vi "Replace Row In File.vi"(9 "Index":i32, 10 "Insert Array":dbl[](array[numeric]), 11 "Path":path) -> (0 "error out":errorcluster)   [LabVIEW 2016]
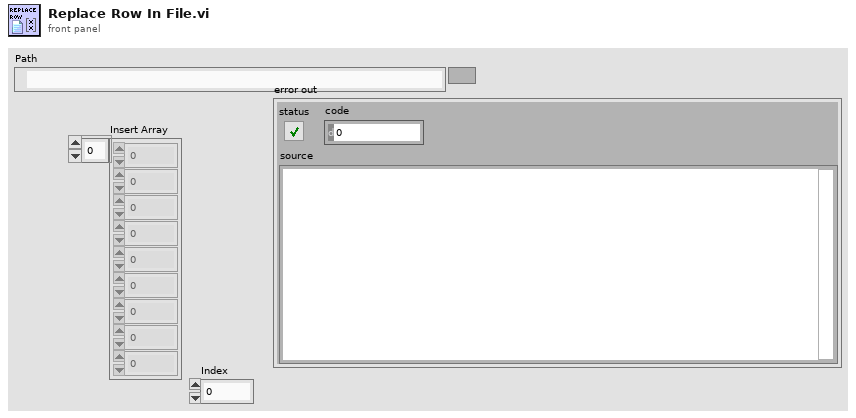
[diagram p1: front panel]
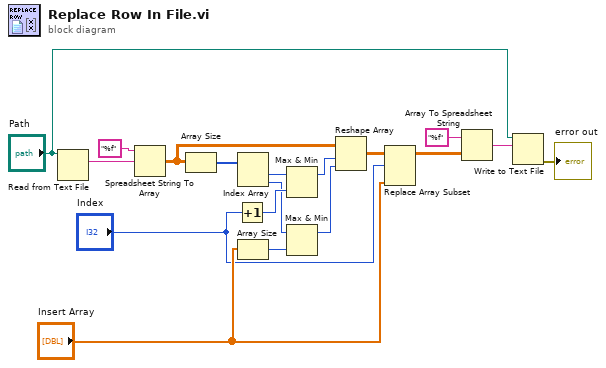
[diagram p0: block diagram]
diagram:
  n1 = Read from Text File(file (use dialog)="Path") -> (text=w15:string)  [unwired: 3 in, 3 out]
  n2 = Spreadsheet String To Array(format string="%f", spreadsheet string=w15) -> (array=w18:dbl[][])  [unwired: 2 in]
  n3 = Array Size(array=w18) -> (size(s)=w11:i32[])
  n4 = Increment(x="Index") -> (x+1=w7:i32)
  n5 = Index Array(array=w11) -> (element #1=w10:i32, element #2=w3:i32)  [unwired: 2 in]
  n6 = Array Size(array="Insert Array") -> (size(s)=w5:i32)
  n7 = Max & Min(x=w10, y=w7) -> (max(x,y)=w9:i32)  [unwired: 1 out]
  n8 = Max & Min(x=w3, y=w5) -> (max(x,y)=w4:i32)  [unwired: 1 out]
  n9 = Reshape Array(w18, w9, w4) -> (w8:dbl[][])
  n10 = Replace Array Subset(array=w8, new element="Insert Array", index (row)="Index") -> (w17:dbl[][])  [unwired: 1 in]
  n11 = Array To Spreadsheet String(array=w17, 3:"%f" ("format string")) -> (spreadsheet string=w14:string)  [unwired: 1 in]
  n12 = Write to Text File(file (use dialog)="Path", text=w14) -> (error out=→"error out":errorcluster)  [unwired: 2 in, 2 out]
